vi "Load and prep N cal images from memory (not file).vi"(10 "default z value":dbl, 11 "data":T1) -> (0 "# of beads":i32, 1 "x,y,(blankz) array":dbl[](array[numeric]), 2 "Array of cal clusters 2":T2(array[cluster]), 3 "cross size":i32, 5 "# slices in stack":i32, 6 "exp/ref array":i32[](array[numeric]))   [LabVIEW 2014]
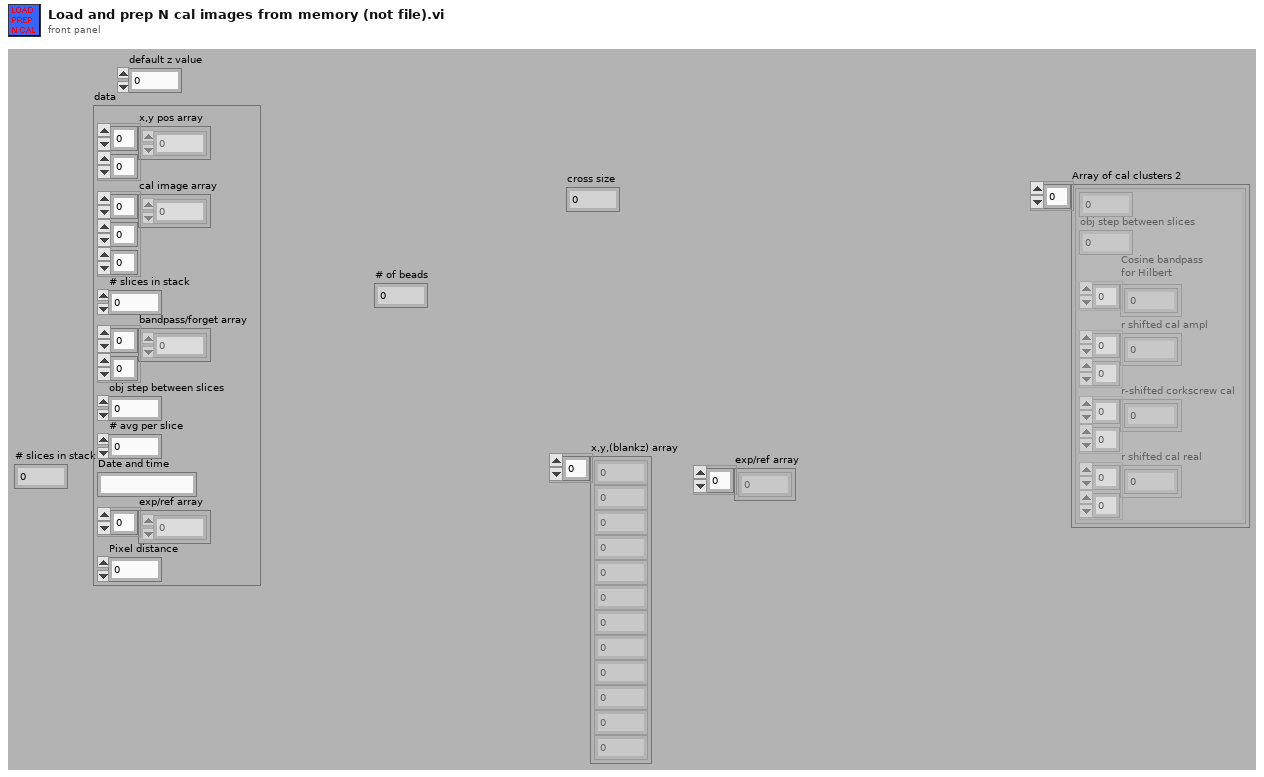
[diagram p1: front panel]
types:
  T1 = cluster{"x,y pos array":dbl[][], "cal image array":dbl[][][], "# slices in stack":i32, "bandpass/forget array":i32[][], "obj step between slices":dbl, "# avg per slice":i32, "Date and time":string, "exp/ref array":i32[], "Pixel distance":dbl}
  T2 = cluster{i32, "obj step between slices":dbl, "Cosine bandpass\nfor Hilbert":dbl[], "r shifted cal ampl":dbl[][], "r-shifted corkscrew cal":cdb[][], "r shifted cal real":dbl[][]}[]
  T3 = cluster{i32, "obj step between slices":dbl, "Cosine bandpass":sgl[], "r shifted cal ampl":dbl[][], "r-shifted corkscrew cal":cdb[][], "r shifted cal real":dbl[][]}
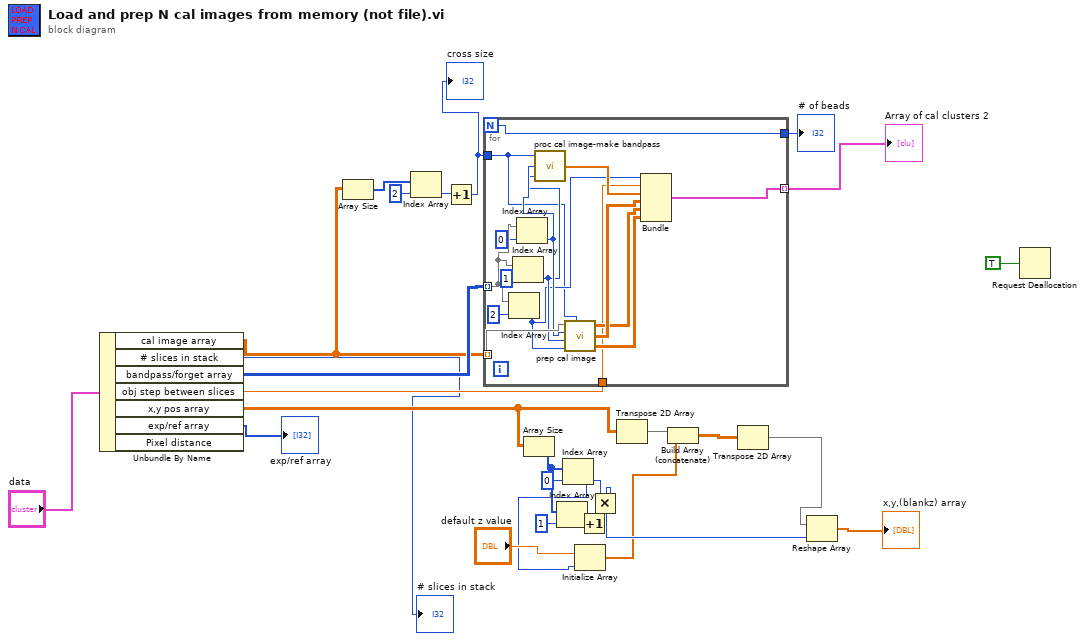
[diagram p0: block diagram]
diagram:
  n1 = Unbundle By Name("data") -> ("cal image array"=w8:dbl[][][], "# slices in stack"=→"# slices in stack":i32, "bandpass/forget array"=w27:i32[][], "obj step between slices"=w26:dbl, "x,y pos array"=w17:dbl[][], "exp/ref array"=→"exp/ref array":i32[])  [unwired: 1 out]
  n2 = Array Size(array=w8) -> (size(s)=w7:i32[])
  n3 = Index Array(array=w7, index=2) -> (element=w5:i32)
  n4 = Increment(x=w5) -> (x+1=w4:i32)
  "cross size" <- w4
  n5 = for {
    N -> [w29]
    tunnel: [w39] -> w2 mode=indexing
    tunnel: w8 -> [w38] mode=indexing
    tunnel: w27 -> [w37] mode=indexing
    tunnel: w26 -> [w31]
    tunnel: [w29] -> w25
    tunnel: w4 -> [w28]
    n6 = Index Array(array=w37, index=2) -> (element=w30:i32)
    n7 = Index Array(array=w37, index=1) -> (element=w32:i32)
    n8 = Index Array(array=w37, index=0) -> (element=w33:i32)
    n9 = call "proc cal image-make bandpass.vi"("HIGH bandpass\n(mode)"=w32, "LOW bandpass\n(mode)"=w33, "# of points (cross size)"=w28) -> ("Cosine bandpass"=w43:sgl[])
    n10 = call "prep cal image.vi"("Raw cal image"=w38, "LOW bandpass\n(mode)"=w33, "HIGH bandpass\n(mode)"=w32, "forget radius"=w30, "# of points (cross size)"=w28) -> ("r-shifted corkscrew cal"=w41:cdb[][], "r shifted cal ampl"=w42:dbl[][], "r shifted cal real"=w40:dbl[][])
    n11 = Bundle(w30, "obj step between slices"=w31, "Cosine bandpass"=w43, "r shifted cal ampl"=w42, "r-shifted corkscrew cal"=w41, "r shifted cal real"=w40) -> (w39:T3)  [unwired: 1 in]
  }
  "# of beads" <- w25
  "Array of cal clusters 2" <- w2
  n12 = Array Size(array=w17) -> (size(s)=w24:i32[])
  n13 = Index Array(array=w24, index=1) -> (element=w21:i32)
  n14 = Index Array(array=w24, index=0) -> (element=w18:i32)
  n15 = Initialize Array("default z value", w18) -> (w16:dbl[])
  n16 = Increment(x=w21) -> (x+1=w14:i32)
  n17 = Multiply(x=w18, y=w14) -> (x*y=w20:i32)
  n18 = Transpose 2D Array(2D array=w17) -> (transposed array=w13:dbl[][])
  n19 = Build Array (concatenate)(w13, w16) -> (w15:dbl[][])
  n20 = Transpose 2D Array(2D array=w15) -> (transposed array=w12:dbl[][])
  n21 = Reshape Array(w12, w20) -> (→"x,y,(blankz) array":dbl[])
  n22 = Request Deallocation(TRUE ("flag")) -> ()
